vi "util_prepare_XY_graph.vi"(4 "Y":dbl format="%#_13g", 6 "X":dbl format="%#_13g", 8 "Y array":dbl[](array[numeric]), 9 "X array":dbl[](array[numeric]), 10 "IsFirst":bool, 11 "XY Graph in":cluster{i32[], dbl[]}[](array[cluster])) -> (0 "Y array out":dbl[](array[numeric]), 1 "X array out":dbl[](array[numeric]), 3 "XY Graph out":cluster{"Array":dbl[], "Array":dbl[]}[](array[cluster]))   [LabVIEW 2020]
doc: "Append an x/y point to a graph."
panel:
  in  "Ignore value":dbl=-1000000.0 format="%#_13g"
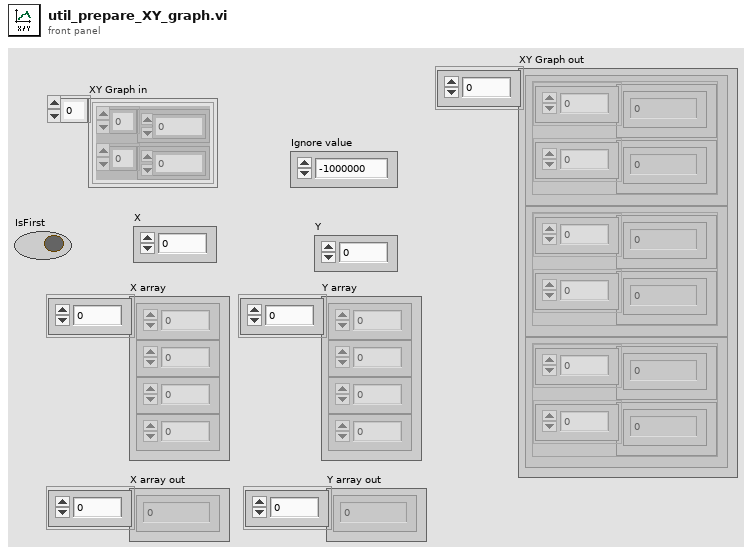
[diagram p1: front panel]
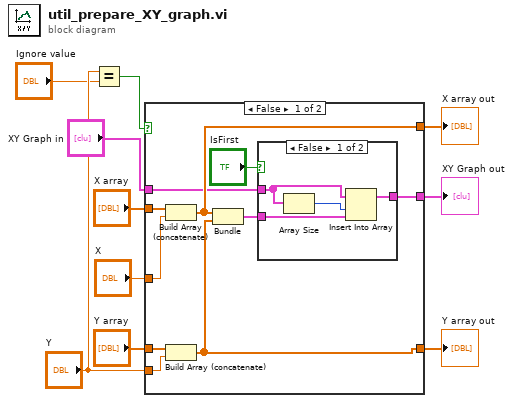
[diagram p0: block diagram]
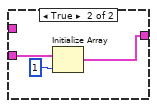
[diagram p2: hidden frame]
diagram:
  n1 = Equal?(x="Y", y="Ignore value") -> (x = y?=w1:bool)
  n2 = case shown="False" w1 {
    tunnel: [w20 w28] -> w10
    tunnel: [w19 w30] -> w9
    tunnel: "X array" -> [w17 w28]
    tunnel: "Y array" -> [w16 w30]
    tunnel: "X" -> [w15 _]
    tunnel: "Y" -> [w14 _]
    tunnel: "XY Graph in" -> [w13 w29]
    tunnel: [w12 w29] -> w4
    frame False {
      n3 = Build Array (concatenate)(w17, w15) -> (w20:dbl[])
      n4 = Build Array (concatenate)(w16, w14) -> (w19:dbl[])
      n5 = Bundle(w20, w19) -> (w18:cluster{dbl[], dbl[]})  [unwired: 1 out]
      n6 = case shown="False" "IsFirst" {
        tunnel: w13 -> [w23 _]
        tunnel: [w22 w25] -> w12
        tunnel: w18 -> [w21 w26]
        frame False {
          n7 = Array Size(array=w23) -> (size(s)=w24:i32)
          n8 = Insert Into Array(array=w23, index=w24, new element=w21) -> (w22:cluster{i32[], dbl[]}[])
        }
        frame True {
          n9 = Initialize Array(w26, 1 ("dimension size")) -> (w25:cluster{dbl[], dbl[]}[])
        }
      }
    }
    frame True {
    }
  }
  "XY Graph out" <- w4
  "Y array out" <- w9
  "X array out" <- w10
